vi "CPP-Equation.vi"(4 "Scan Period":dbl format="%.2f", 5 "Previous Scan Value":dbl format="%.2f", 6 "Present scan array":dbl[](array[numeric]) format="%.2f", 7 "Value to Output":dbl format="%.2f", 8 "Ch Description":T1={"Ch Name"="Tunnel3:Pressures:", "Type"="", "Function"=enum."Analogue Input", "Ch State"=enum."On", "Calibration type"="", "A"=30.0, "B"=10.0, "C"=0.0, "D"=0.0, "Comments"="", "Address"={"Main"=0, "Ch."=0, "Sub"=0, "Port Name"=""}, "String"="", "Duty"=65535} {"Duty" format="%016b"; "D" format="%#_5g"; "C" format="%#_5g"; "B" format="%#_5g"; "A" format="%#_5g"}, 9 "Ch names":string[](array[string])) -> (0 "Scan comment":string, 1 "Output":dbl=0.0037402657506766107 format="%.4g", 3 "HelpText":string="\"A\" Warn if above this value\n\"B\" Warn if below this value\n\"C\" Hysteresis margin\n\"D\" is the averaging time in minutes\n\nWrite Channel name to check in the box above \"Comparator\"")   [LabVIEW 2016]
doc: "Wrapper for CPP-ZerosMaintenance.vi\nChannels Names should have the format \"Tunnel#:Pressures:\" (e.g. Tunnel1:Pressures: or Tunnel3:Pressures:). A = SecondsToMonitor (intervall to determine if tunnel has been off long enough and to inspect zero drift. B = SecondsToAverage (averaging interval for transducer zeros)."
uses:
  ADAM Client/Sub VIs/ADAM Controls/Ch_description_ADAM.ctl
  ADAM Client/Sub VIs/ADAM Controls/Module_type_ADAM.ctl
  ADAM Client/Sub VIs/ADAM Controls/Function_ADAM.ctl
  ADAM Client/Sub VIs/ADAM Controls/Channel_State.ctl
  ADAM Client/Sub VIs/ADAM Controls/Calib_type_ADAM.ctl
  ADAM Client/Sub VIs/ADAM Controls/Address.ctl
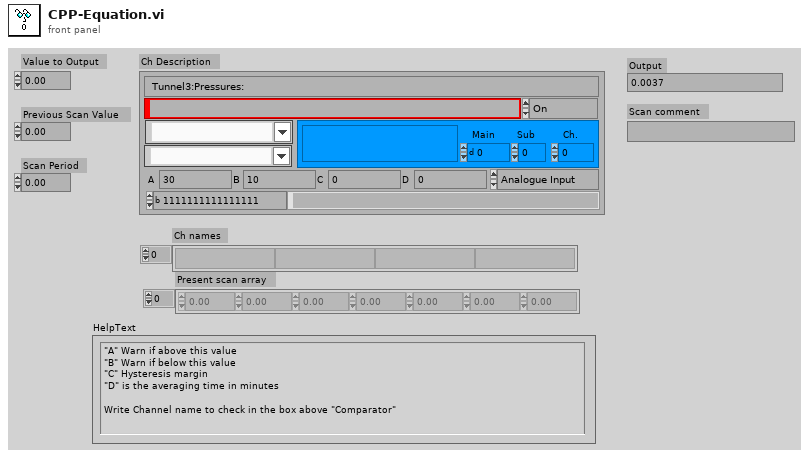
[diagram p1: front panel]
types:
  T1 = typedef "Ch_description_ADAM.ctl" = cluster{"Ch Name":string, "Type":T2, "Function":T3, "Ch State":T4, "Calibration type":T5, "A":dbl, "B":dbl, "C":dbl, "D":dbl, "Comments":string, "Address":T6, "String":string, "Duty":u16}
  T2 = typedef "Module_type_ADAM.ctl" = string
  T3 = typedef "Function_ADAM.ctl" = enum16{"Analogue Input", "Digital Input", "Event counter", "Event rate", "Analogue Output", "Digital Output", "Relay Output"}
  T4 = typedef "Channel_State.ctl" = enum16{"On", "Off", "Always On", "Always Off"}
  T5 = typedef "Calib_type_ADAM.ctl" = string
  T6 = typedef "Address.ctl" = cluster{"Main":i32, "Ch.":i32, "Sub":i32, "Port Name":string}
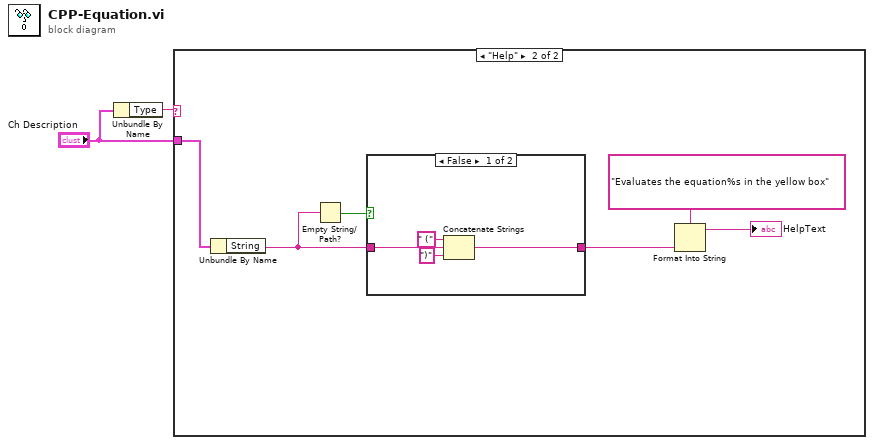
[diagram p0: block diagram]
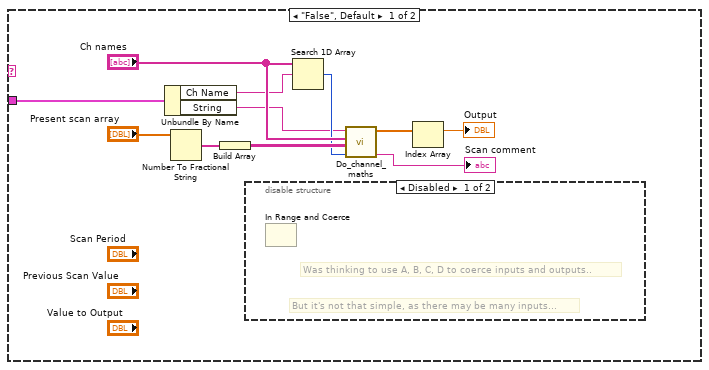
[diagram p2: hidden frame]
diagram:
  n1 = Unbundle By Name("Ch Description") -> ("Type"=w1:T2)
  n2 = case shown="\"Help\"" w1 {
    tunnel: "Ch Description" -> [w13 w19]
    frame "False", Default {
      n3 = Unbundle By Name(w13) -> ("Ch Name"=w6:string, "String"=w7:string)
      n4 = Number To Fractional String(number="Present scan array") -> (F-format string=w12:string[])  [unwired: 3 in]
      n5 = Build Array(w12) -> (w11:string[][])
      n6 = disable-structure shown="Disabled" {
        frame Disabled {
          # "But it's not that simple, as there may be many inputs..."
          # "Was thinking to use A, B, C, D to coerce inputs and outputs.."
          n7 = In Range and Coerce() -> ()  [unwired: 3 in, 2 out]
        }
        frame Enabled {
        }
      }
      n8 = Search 1D Array(1D array="Ch names", element=w6) -> (index of element=w8:i32)  [unwired: 1 in]
      n9 = call "Do_channel_maths.vi"("Output Index"=w8, "Channel Values In"=w11, "Channel Names"="Ch names", "Maths Equation"=w7) -> ("Error String"=→"Scan comment":string, "Results"=w5:dbl[])  [unwired: 1 in, 1 out]
      n10 = Index Array(array=w5) -> (element=→"Output":dbl)  [unwired: 1 in]
    }
    frame "Help" {
      n11 = Unbundle By Name(w19) -> ("String"=w15:string)
      n12 = Empty String/Path?(string/path=w15) -> (empty?=w16:bool)
      n13 = case shown="False" w16 {
        tunnel: [w22 w24] -> w17
        tunnel: w15 -> [w23 w24]
        frame False {
          n14 = Concatenate Strings(" (" ("string"), w23, ")" ("string")) -> (w22:string)
        }
        frame True {
        }
      }
      n15 = Format Into String(format string="Evaluates the equation%s in the yellow box", w17) -> (resulting string=→"HelpText":string)  [unwired: 2 in, 1 out]
    }
  }
